vi "delete_zeros_new.vi"(11 "Array in":dbl[](array[numeric])) -> (3 "Array out":dbl[](array[numeric]))   [LabVIEW 2018]
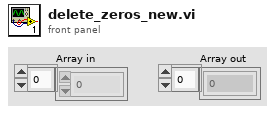
[diagram p1: front panel]
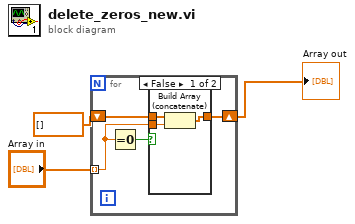
[diagram p0: block diagram]
diagram:
  n1 = for {
    shift-right: [w4] -> w2
    shift-left: dbl[] [] -> [w6]
    tunnel: "Array in" -> [w5] mode=indexing
    n2 = Equal To 0?(x=w5) -> (x = 0?=w7:bool)
    n3 = case shown="False" w7 {
      tunnel: w6 -> [w10 w11]
      tunnel: w5 -> [w9 _]
      tunnel: [w8 w11] -> w4
      frame False {
        n4 = Build Array (concatenate)(w10, w9) -> (w8:dbl[])
      }
      frame True {
      }
    }
  }
  "Array out" <- w2
